vi "Read Host.vi"(8 "error in (no error)":errorcluster, 11 "Host":T1) -> (0 "error out":errorcluster, 2 "Host":T2, 3 "Host out":T1)   [LabVIEW 2013, in "libssh2.lvlib"]
uses:
  libssh2.lvlib
  libssh2_knownhost.ctl
  Host Refnum.ctl
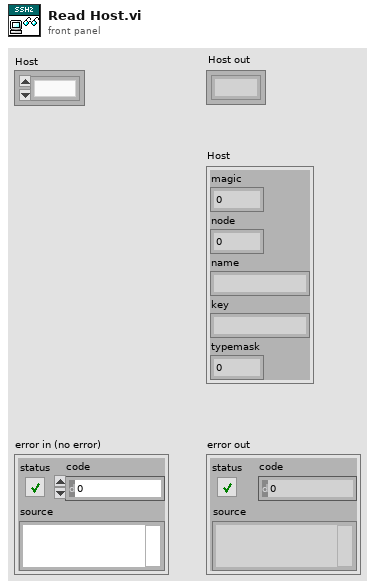
[diagram p1: front panel]
types:
  T1 = typedef "libssh2.lvlib/Host Refnum.ctl" = refnum<k1>
  T2 = typedef "libssh2.lvlib/libssh2_knownhost.ctl" = cluster{"magic":u32, "node":u64, "name":string, "key":string, "typemask":i32}
  T3 = cluster{"magic":u32, "node":u64, "name":u64, "key":u64, "typemask":i32}
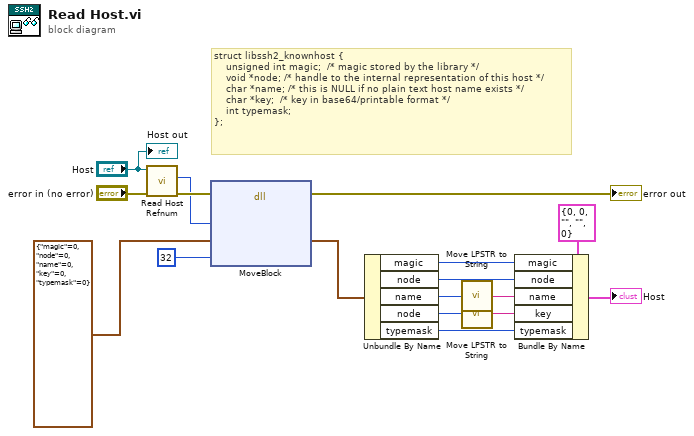
[diagram p0: block diagram]
diagram:
  # "struct libssh2_knownhost {\n    unsigned int magic;  /* magic stored by the library */\n    void *node; /* handle to the internal representation of this host */\n    char *name; /* this is NULL if no plain text host name exists */\n    char *key;  /* key in base64/printable format */\n    int typemask;\n};"
  n1 = call "Read Host Refnum.vi"("error in (no error)"="error in (no error)", "Host"="Host") -> ("error out"=w14:errorcluster, "libssh2_knownhost*"=w11:u64)  [unwired: 8 in]
  n2 = dll-call lib="LabVIEW" fn="MoveBlock"(error in=w14, "ps"=w11, T3 {"magic"=0, "node"=0, "name"=0, "key"=0, "typemask"=0}, "size"=i64 32) -> (error out=→"error out":errorcluster, w8:T3)  [unwired: 5 in, 1 out]
  n3 = Unbundle By Name(w8) -> ("magic"=w6:u32, "node"=w5:u64, "name"=w7:u64, "node"=w3:u64, "typemask"=w1:i32)
  n4 = call "Move LPSTR to String.vi"("LPSTR"=w7) -> ("String"=w4:string)  [unwired: 1 in]
  n5 = call "Move LPSTR to String.vi"("LPSTR"=w3) -> ("String"=w2:string)  [unwired: 1 in]
  n6 = Bundle By Name(cluster=T2 {"magic"=0, "node"=0, "name"="", "key"="", "typemask"=0} ("libssh2_knownhost"), "magic"=w6, "node"=w5, "name"=w4, "key"=w2, "typemask"=w1) -> (→"Host":T2)
  "Host out" <- "Host"
